vi "Cross Power Spectrum.vi"(3 "dt":dbl=1.0 format="%0.2f", 4 "Signal Y (V)":dbl[](array[numeric]), 5 "Signal X (V)":dbl[](array[numeric])) -> (0 "df":dbl format="%#.6g", 1 "Cross Power XY Spectrum Phase (radians)":dbl[](array[numeric]), 2 "Cross Power XY Spectrum Mag (V^2rms)":dbl[](array[numeric]))   [LabVIEW 2020, in "NI_AALPro.lvlib"]
doc: "Computes the single-sided, scaled, cross power spectrum of two real-time signals."
uses:
  <vilib>/Analysis/NI_AALPro.lvlib
  <vilib>/Analysis/2dsp.llb/Cross Power (DBL).vi
panel:
  # "Cross Power Spectrum"
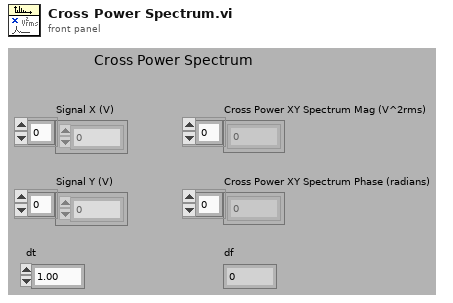
[diagram p1: front panel]
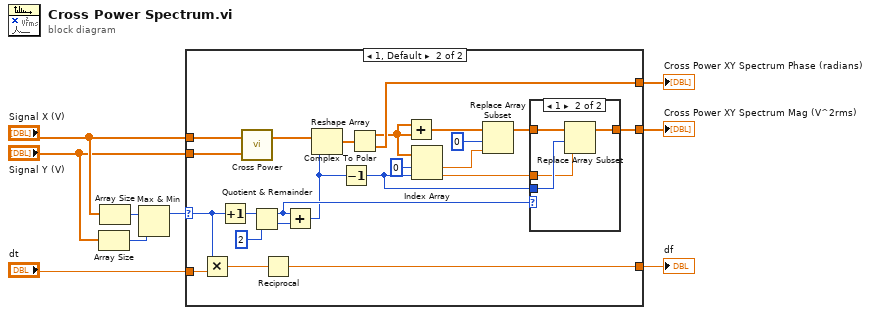
[diagram p0: block diagram]
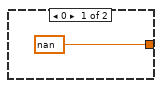
[diagram p2: hidden frame]
diagram:
  n1 = Array Size(array="Signal Y (V)") -> (size(s)=w4:i32)
  n2 = Array Size(array="Signal X (V)") -> (size(s)=w5:i32)
  n3 = Max & Min(x=w5, y=w4) -> (max(x,y)=w1:i32)  [unwired: 1 out]
  n4 = case shown="1, Default" w1 {
    selector: w1 -> [_ w11]
    tunnel: "dt" -> [_ w32]
    tunnel: [nan w31] -> w8
    tunnel: [_ w30] -> w7
    tunnel: "Signal X (V)" -> [_ w25]
    tunnel: "Signal Y (V)" -> [_ w24]
    tunnel: [_ w17] -> w2
    frame 0 {
    }
    frame 1, Default {
      n5 = Multiply(x=w11, y=w32) -> (x*y=w33:dbl)
      n6 = Increment(x=w11) -> (x+1=w23:i32)
      n7 = call-poly <vilib>:"Cross Power.vi"("Y"=w24, "X"=w25) -> ("Sxy"=w14:cdb[])  [unwired: 1 out]
      n8 = Quotient & Remainder(x=w23, y=2) -> (x-y*floor(x/y)=w19:i32, floor(x/y)=w22:i32)
      n9 = Reciprocal(x=w33) -> (1/x=w31:dbl)
      n10 = Add(x=w19, y=w22) -> (x+y=w12:i32)
      n11 = Reshape Array(w14, w12) -> (w13:cdb[])
      n12 = Decrement(x=w12) -> (x-1=w15:i32)
      n13 = Complex To Polar(r * e^(i*theta)=w13) -> (r=w29:dbl[], theta=w30:dbl[])
      n14 = Add(x=w29, y=w29) -> (x+y=w28:dbl[])
      n15 = Index Array(array=w29, index #1=0 ("index"), index #2=w15) -> (element #1=w27:dbl, element #2=w16:dbl)
      n16 = Replace Array Subset(array=w28, new element=w27, index=0) -> (w18:dbl[])
      n17 = case shown="1" w19 {
        tunnel: w18 -> [w34 w37]
        tunnel: [w34 w38] -> w17
        tunnel: w16 -> [_ w35]
        tunnel: w15 -> [_ w36]
        frame 0, Default {
        }
        frame 1 {
          n18 = Replace Array Subset(array=w37, new element=w35, index=w36) -> (w38:dbl[])
        }
      }
    }
  }
  "Cross Power XY Spectrum Mag (V^2rms)" <- w2
  "Cross Power XY Spectrum Phase (radians)" <- w7
  "df" <- w8
